vi "Update ClockID.vi"(8 "error in (no error)":errorcluster, 10 "ClockID":u8, 11 "CIFChannelMng in":refnum<class "CIFChannelMng.lvclass">) -> (0 "error out":errorcluster, 3 "CIFChannelMng out":refnum<class "CIFChannelMng.lvclass">)   [LabVIEW 2021, in "CIFChannelMng.lvclass"]
uses:
  CIFChannelMng.lvclass
  CIFChannelMng.lvclass/CIFChannelMng.ctl
  CIFChannels/CIFChannels.lvclass
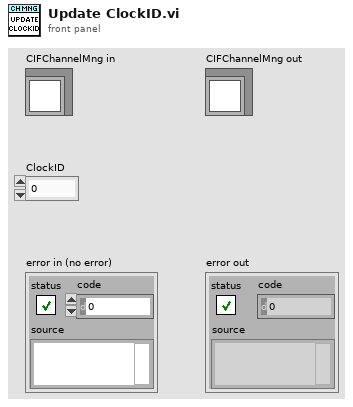
[diagram p1: front panel]
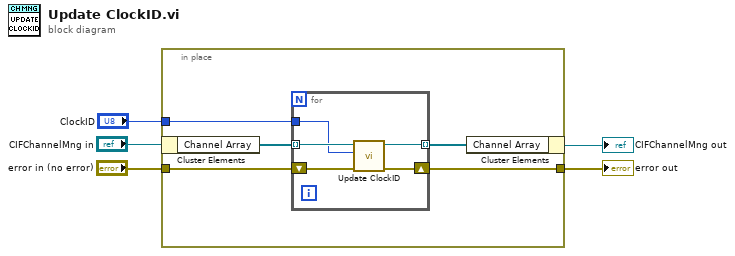
[diagram p0: block diagram]
diagram:
  n1 = in-place {
    in-place-border: "error in (no error)" -> [w9]
    in-place-border: "ClockID" -> [w8]
    in-place-border: [w6] -> w1
    n2 = in-place-cluster #1("CIFChannelMng in") -> ("Channel Array"=w10:refnum<class "CIFChannels.lvclass">[])
    n3 = for {
      tunnel: w10 -> [w15] mode=indexing
      tunnel: w8 -> [w13]
      tunnel: [w12] -> w7 mode=indexing
      shift-right: [w11] -> w6
      shift-left: w9 -> [w14]
      n4 = call-dynamic "Update ClockID.vi"("error in (no error)"=w14, "ClockID"=w13, "CIFChannels in"=w15) -> ("error out"=w11:errorcluster, "CIFChannels out"=w12:refnum<class "CIFChannels.lvclass">)  [unwired: 7 in]
    }
    n5 = in-place-cluster #1("Channel Array"=w7) -> (→"CIFChannelMng out":refnum<class "CIFChannelMng.lvclass">)
  }
  "error out" <- w1
